vi "PC_DCG_Single.vi"() -> ()   [LabVIEW 2021]
uses:
  Digital Clock Generation/Typedefs/Digital Clock Settings.ctl
  Digital Clock Generation/Typedefs/Actual Clock Settings.ctl
  Digital Clock Generation/DAQ_Digital Clock Generation.lvlib
panel:
  out "error out":errorcluster
  out "Actual Clock Settings":T1={"Frequency (Hz)"=10000.0, "Duty Cycle (%)"=50.0, "Generation Time (s)"=0.1} {"Duty Cycle (%)" format="%#.2p"; "Frequency (Hz)" format="%.6p"; "Generation Time (s)" format="%.2p"}
  in  "Digital Clock Settings":T2={"Frequency (Hz)"=10000.0, "Duty Cycle(%)"=50.0, "Generation Time (s)"=0.1} {"Duty Cycle(%)" format="%#.2p"; "Frequency (Hz)" format="%.6p"; "Generation Time (s)" format="%.2p"}
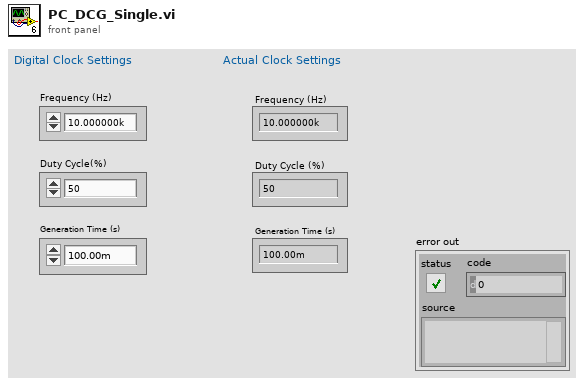
[diagram p1: front panel]
types:
  T1 = typedef "DAQ_Digital Clock Generation.lvlib/Actual Clock Settings.ctl" = cluster{"Frequency (Hz)":dbl, "Duty Cycle (%)":dbl, "Generation Time (s)":dbl}
  T2 = typedef "DAQ_Digital Clock Generation.lvlib/Digital Clock Settings.ctl" = cluster{"Frequency (Hz)":dbl, "Duty Cycle(%)":dbl, "Generation Time (s)":dbl}
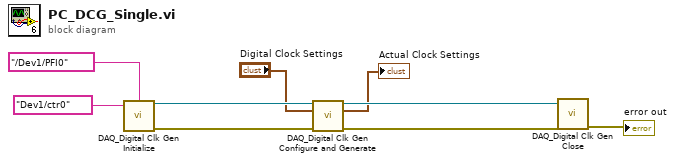
[diagram p0: block diagram]
diagram:
  n1 = call "DAQ_Digital Clk Gen Initialize.vi"("Physical Channel (Counter)"=tag "Dev1/ctr0", "Output Terminal"=tag "/Dev1/PFI0") -> ("DAQmx Task Out"=w7:refnum<k21>, "error out"=w3:errorcluster)  [unwired: 12 in]
  n2 = call "DAQ_Digital Clk Gen Configure and Generate.vi"("DAQmx Task In"=w7, "Digital Clock Settings"="Digital Clock Settings", "error in"=w3) -> ("DAQmx Task Out"=w6:refnum<k21>, "Actual Clock Settings"=→"Actual Clock Settings":T1, "error out"=w2:errorcluster)  [unwired: 10 in]
  n3 = call "DAQ_Digital Clk Gen Close.vi"("DAQmx Task In"=w6, "error in"=w2) -> ("error out"=→"error out":errorcluster)  [unwired: 13 in]
